vi "subGetWiiMoteState(AccelButtonsIR).vi"(0 "Wiimote":refnum<k24>, 1 "error in":errorcluster) -> (2 "reference out":refnum<k24>, 3 "Wiimote State":T2, 4 "IRState":T1 {"Mode" items=["Off"=0, "Basic"=1, "Extended"=3, "Full"=5]}, 5 "error out":errorcluster)   [LabVIEW 2010]
doc: "Get accel / button state from wiimote \nSam Shearman"
uses:
  wiimotestate.ctl
  C:/Users/×ñÞóôïò/Desktop/rtdsp_project14_4_11/3D_Experiment/libs/ola/WiimoteManaged(wml17)/WiimoteLib.dll
  WiimoteLib.dll
  wiimoteState(IR).ctl
panel:
  # "Establish a Bluetooth link with your Wiimote prior to executing this VI.\n\nRequires the Wiimote Managed Library WiimoteLib Ver 1.7\navailable from http://www.codeplex.com/WiimoteLib\nSam Shearman"
  # "Accelerometers"
  # "Buttons"
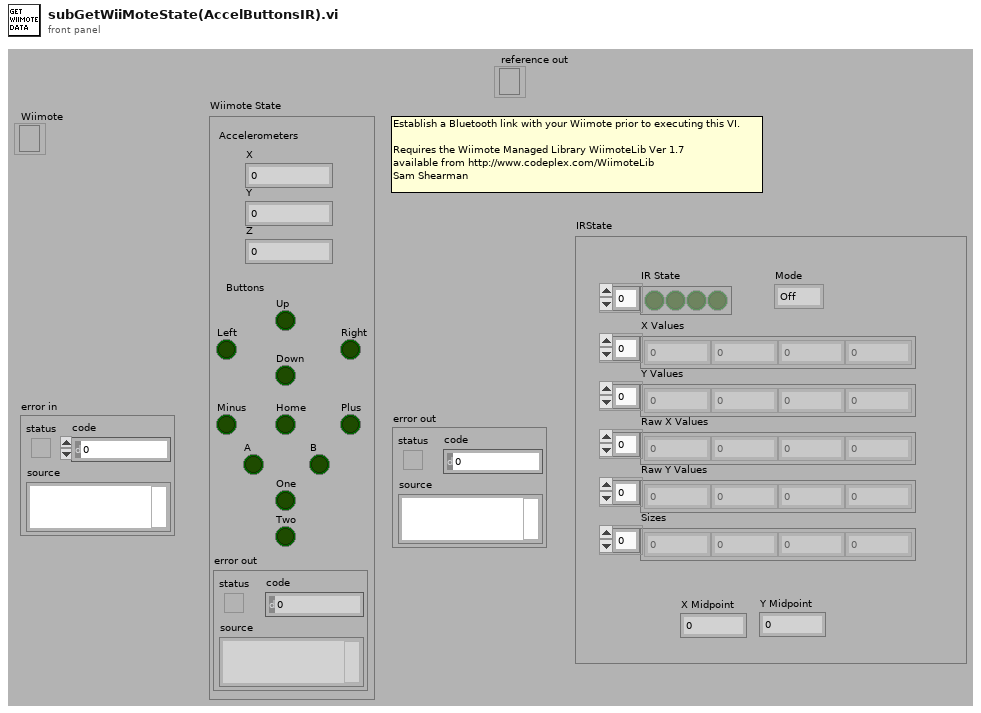
[diagram p1: front panel]
types:
  T1 = typedef "wiimoteState(IR).ctl" = cluster{"Mode":u8, "IR State":bool[], "X Values":sgl[], "Y Values":sgl[], "Raw X Values":i32[], "Raw Y Values":i32[], "Sizes":i32[], "X Midpoint":sgl, "Y Midpoint":sgl}
  T2 = typedef "wiimotestate.ctl" = cluster{"X":sgl, "Y":sgl, "Z":sgl, "A":bool, "B":bool, "Down":bool, "Home":bool, "Left":bool, "Minus":bool, "One":bool, "Plus":bool, "Right":bool, "Two":bool, "Up":bool, "error out":errorcluster}
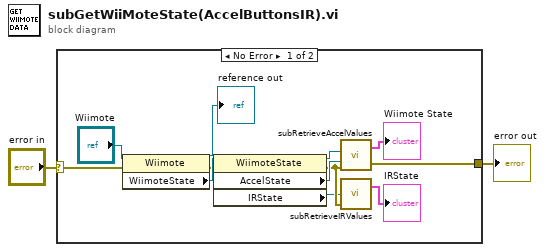
[diagram p0: block diagram]
diagram:
  n1 = case shown="No Error" "error in" {
    selector: "error in" -> [w7 w15]
    tunnel: [w6 w15] -> w2
    frame No Error {
      n2 = property class="Wiimote"(reference="Wiimote", error in=w7) -> (reference out=→"reference out":refnum<k24>, error out=w11:errorcluster, "WiimoteState"=w12:refnum<k24>)
      n3 = property class="WiimoteState"(reference=w12, error in=w11) -> (reference out=w9:refnum<k24>, error out=w4:errorcluster, "AccelState"=w13:refnum<k24>, "IRState"=w3:refnum<k24>)
      n4 = call "subRetrieveAccelValues.vi"("error in"=w4, "AccelState"=w13, "WiimoteState"=w9) -> ("error out"=w6:errorcluster, "Wiimote State"=→"Wiimote State":T2)  [unwired: 1 out]
      n5 = call "subRetrieveIRValues.vi"("error in"=w4, "IRState"=w3) -> ("IRState"=→"IRState":T1)  [unwired: 1 in, 1 out]
    }
    frame Error {
    }
  }
  "error out" <- w2
